vi "Stop.vi"(8 "error in (no error)":errorcluster, 11 "AlphaStep One in":refnum<class "AlphaStep One.lvclass">) -> (0 "error out":errorcluster, 3 "AlphaStep One out":refnum<class "AlphaStep One.lvclass">)   [LabVIEW 2015, in "AlphaStep One.lvclass"]
uses:
  AlphaStep One.lvclass
  AlphaStep One.lvclass/AlphaStep One.ctl
  Serial Device/Serial Device.lvclass
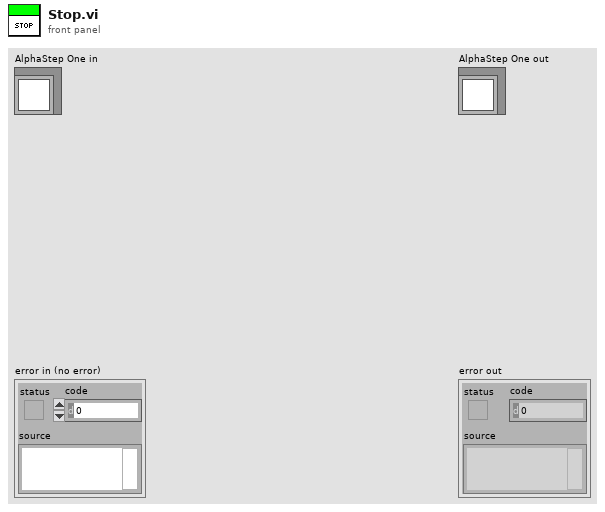
[diagram p1: front panel]
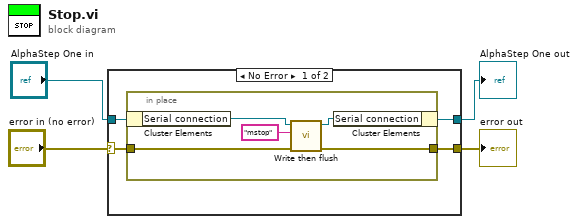
[diagram p0: block diagram]
diagram:
  n1 = case shown="No Error" "error in (no error)" {
    selector: "error in (no error)" -> [w6 w14]
    tunnel: "AlphaStep One in" -> [w8 w15]
    tunnel: [w7 w15] -> w2
    tunnel: [w5 w14] -> w1
    frame No Error {
      n2 = in-place {
        in-place-border: w6 -> [w11]
        in-place-border: [w10] -> w5
        n3 = in-place-cluster #1(w8) -> ("Serial connection"=w13:refnum<class "Serial Device.lvclass">)
        n4 = call "Write then flush.vi"("error in (no error)"=w11, "TX Data"="mstop", "Serial Device in"=w13) -> ("error out"=w10:errorcluster, "Serial Device out"=w9:refnum<class "Serial Device.lvclass">)  [unwired: 7 in]
        n5 = in-place-cluster #1("Serial connection"=w9) -> (w7:refnum<class "AlphaStep One.lvclass">)
      }
    }
    frame Error {
    }
  }
  "error out" <- w1
  "AlphaStep One out" <- w2
